vi "Read Listener Port Ref.vi"(8 "error in (no error)":errorcluster, 11 "Listener in":refnum<class "Listener.lvclass">) -> (0 "error out":errorcluster, 2 "Listener Port Ref":refnum<visa-resource-name>, 3 "Listener out":refnum<class "Listener.lvclass">)   [LabVIEW 2018, in "Listener.lvclass"]
uses:
  Listener.lvclass
  Listener.lvclass/Listener.ctl
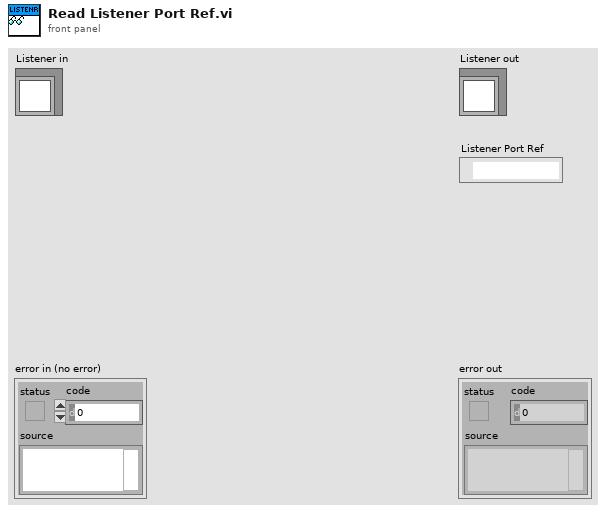
[diagram p1: front panel]
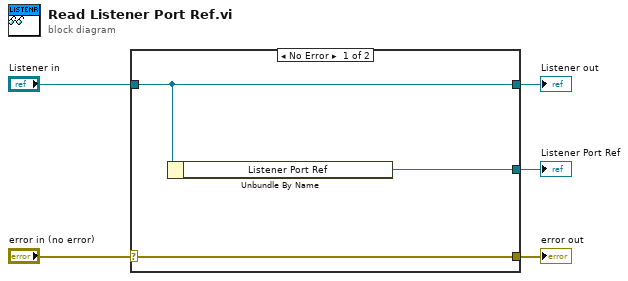
[diagram p0: block diagram]
diagram:
  n1 = case shown="No Error" "error in (no error)" {
    selector: "error in (no error)" -> [w8 w9]
    tunnel: [w8 w9] -> w4
    tunnel: [w7 w10] -> w2
    tunnel: "Listener in" -> [w7 w10]
    tunnel: [w6 _] -> w1
    frame No Error {
      n2 = Unbundle By Name(w7) -> ("Listener Port Ref"=w6:refnum<visa-resource-name>)
    }
    frame Error {
    }
  }
  "error out" <- w4
  "Listener out" <- w2
  "Listener Port Ref" <- w1
